vi "Get DIO Bits to Execute Stored Program Status.vi"(4 "error in (no error)":errorcluster, 7 "VISA resource name":refnum<visa-resource-name>) -> (0 "error out":errorcluster, 2 "Program Name":string, 3 "VISA resource name out":refnum<visa-resource-name>)   [LabVIEW 2019, in "Newport ESP301.lvlib"]
doc: "Reports the current setting about assigned DIO bits to execute stored programs."
uses:
  Newport ESP301.lvlib
panel:
  in  "Bit Number (0)":i32 min=0 max=15
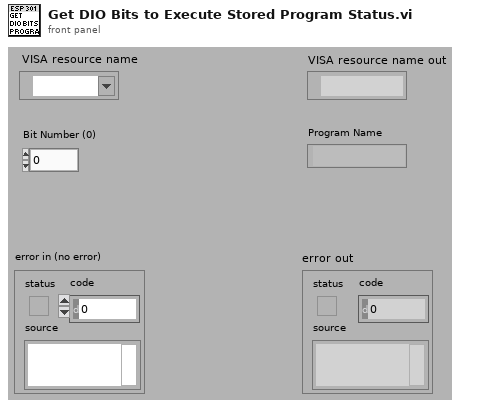
[diagram p1: front panel]
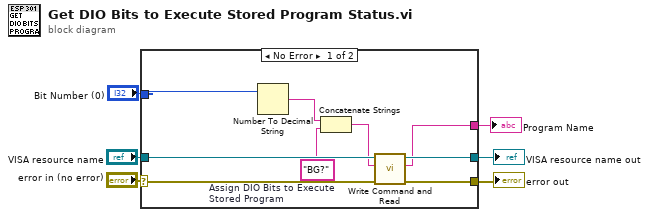
[diagram p0: block diagram]
diagram:
  n1 = case shown="No Error" "error in (no error)" {
    selector: "error in (no error)" -> [w12 w17]
    tunnel: [w14 w17] -> w6
    tunnel: "VISA resource name" -> [w15 w16]
    tunnel: [w13 w16] -> w5
    tunnel: [w11 _] -> w2
    tunnel: "Bit Number (0)" -> [w10 _]
    frame No Error {
      w8 = "BG?"  # Assign DIO Bits to Execute Stored Program
      n2 = Number To Decimal String(number=w10) -> (decimal integer string=w9:string)  [unwired: 1 out]
      n3 = Concatenate Strings(w9, w8) -> (w7:string)
      n4 = call "Write Command and Read.vi"("error in (no error)"=w12, "Command"=w7, "VISA resource name"=w15) -> ("error out"=w14:errorcluster, "Returned string"=w11:string, "VISA resource name out"=w13:refnum<visa-resource-name>)  [unwired: 2 in, 2 out]
    }
    frame Error {
    }
  }
  "error out" <- w6
  "VISA resource name out" <- w5
  "Program Name" <- w2
